vi "get_rpm.vi"(2 "error in (no error)":errorcluster) -> (0 "RPM":dbl, 1 "error out":errorcluster)   [LabVIEW 2019]
uses:
  rpm.vi
  <vilib>/Analysis/NI_AALBase.lvlib
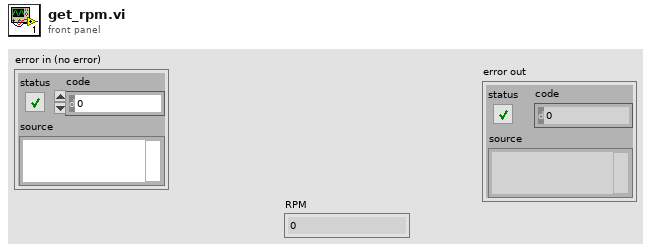
[diagram p1: front panel]
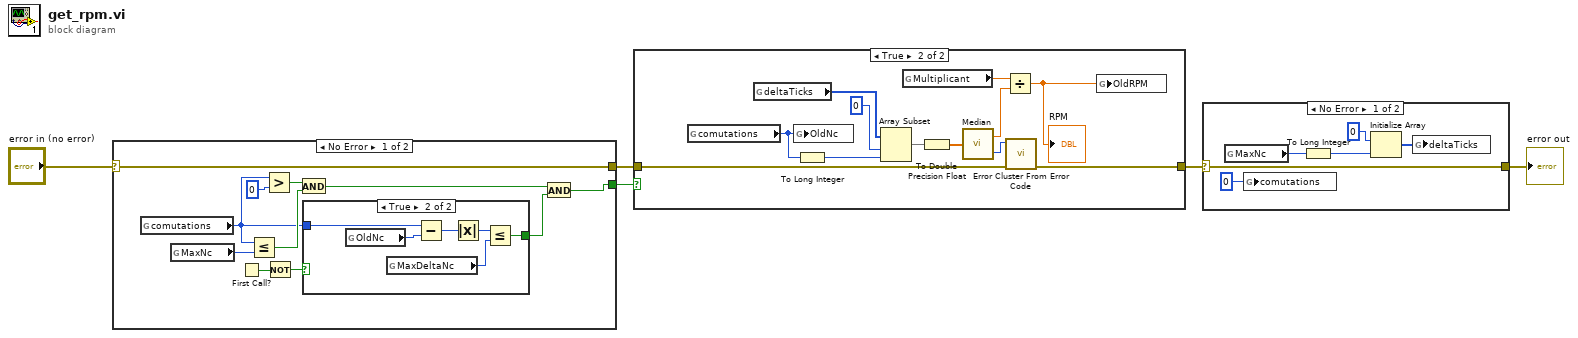
[diagram p0: block diagram]
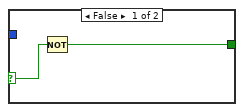
[diagram p2: hidden frame]
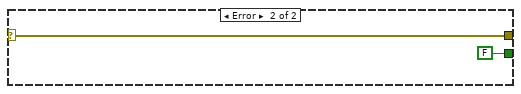
[diagram p3: hidden frame]
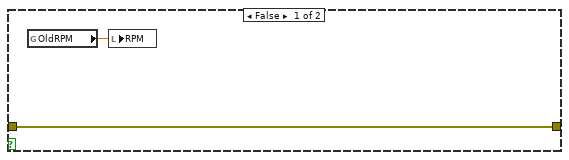
[diagram p4: hidden frame]
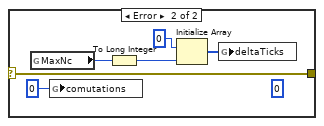
[diagram p5: hidden frame]
diagram:
  n1 = case shown="No Error" "error in (no error)" {
    selector: "error in (no error)" -> [w6 w26]
    tunnel: [w12 FALSE] -> w3
    tunnel: [w6 w26] -> w2
    frame No Error {
      n2 = global read "rpm.vi" "comutations"() -> (w10:i64)
      n3 = global read "rpm.vi" "MaxNc"() -> (w13:i64)
      n4 = First Call?() -> (First Call?: T/F=w8:bool)
      n5 = Less Or Equal?(x=w10, y=w13) -> (x <= y?=w14:bool)
      n6 = Greater?(x=w10, y=i64 0) -> (0:w15:bool)
      n7 = Not(x=w8) -> (.not. x?=w7:bool)
      n8 = And(x=w15, y=w14) -> (x .and. y?=w11:bool)
      n9 = case shown="True" w7 {
        selector: w7 -> [w18 _]
        tunnel: w10 -> [_ w24]
        tunnel: [w17 w22] -> w9
        frame False {
          n10 = Not(x=w18) -> (.not. x?=w17:bool)
        }
        frame True {
          n11 = global read "rpm.vi" "OldNc"() -> (w23:i64)
          n12 = global read "rpm.vi" "MaxDeltaNc"() -> (w19:i64)
          n13 = Subtract(x=w24, y=w23) -> (x-y=w20:i64)
          n14 = Absolute Value(x=w20) -> (abs(x)=w21:i64)
          n15 = Less Or Equal?(x=w21, y=w19) -> (x <= y?=w22:bool)
        }
      }
      n16 = And(x=w11, y=w9) -> (x .and. y?=w12:bool)
    }
    frame Error {
    }
  }
  n17 = case shown="True" w3 {
    tunnel: w2 -> [w27 w33]
    tunnel: [w27 w31] -> w4
    frame False {
      n18 = global read "rpm.vi" "OldRPM"() -> (w28:dbl)
      n19 = local write "RPM"(w28) -> ()
    }
    frame True {
      n20 = global read "rpm.vi" "comutations"() -> (w30:i64)
      n21 = global read "rpm.vi" "deltaTicks"() -> (w40:i64[])
      n22 = global write "rpm.vi" "OldNc"(w30) -> ()
      n23 = To Long Integer(number=w30) -> (32bit integer=w29:i32)
      n24 = Array Subset(array=w40, index=0, length=w29) -> (w38:i64[])
      n25 = global read "rpm.vi" "Multiplicant"() -> (w35:dbl)
      n26 = To Double Precision Float(number=w38) -> (double precision float=w37:dbl[])
      n27 = call <vilib>:"Median.vi"("X"=w37) -> ("median"=w34:dbl, "error"=w32:i32)
      n28 = Divide(x=w35, y=w34) -> (x/y=w36:dbl)
      "RPM" <- w36
      n29 = call <vilib>:"Error Cluster From Error Code.vi"("error in (no error)"=w33, "error code (0)"=w32) -> ("error out"=w31:errorcluster)  [unwired: 7 in]
      n30 = global write "rpm.vi" "OldRPM"(w36) -> ()
    }
  }
  n31 = case shown="No Error" w4 {
    selector: w4 -> [w46 w52]
    tunnel: [w46 w52] -> w5
    frame No Error {
      n32 = global read "rpm.vi" "MaxNc"() -> (w43:i64)
      n33 = global write "rpm.vi" "comutations"(i64 0 ("comutations")) -> ()
      n34 = To Long Integer(number=w43) -> (32bit integer=w41:i32)
      n35 = Initialize Array(i64 0, w41) -> (w44:i64[])
      n36 = global write "rpm.vi" "deltaTicks"(w44) -> ()
    }
    frame Error {
      (unwired) i64 0
      n37 = global read "rpm.vi" "MaxNc"() -> (w50:i64)
      n38 = global write "rpm.vi" "comutations"(i64 0 ("comutations")) -> ()
      n39 = To Long Integer(number=w50) -> (32bit integer=w49:i32)
      n40 = Initialize Array(i64 0 ("element"), w49) -> (w48:i64[])
      n41 = global write "rpm.vi" "deltaTicks"(w48) -> ()
    }
  }
  "error out" <- w5
